vi "lvssh2_session_callback_send_32.vi"(4 "lvssh2_session_callback_send_function":refnum<vi>, 5 "Event Data":T1, 6 "User Event Ref":refnum<user-event>, 7 "Event Common Data":T3 {"Event Source" items=["LabVIEW UI"=0, "ActiveX"=1, "User Event"=25]}) -> ()   [LabVIEW 2013, in "libssh2.lvlib"]
uses:
  libssh2.lvlib
  <vilib>/event_ctls.llb/eventsource.ctl
  lvssh2_session_callback_send_function_input_args_32.ctl
  lvssh2_extensions.dll
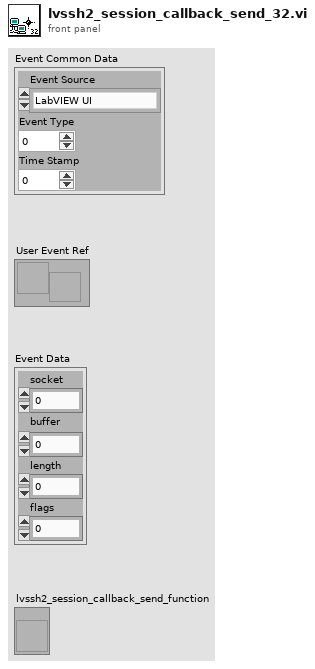
[diagram p1: front panel]
types:
  T1 = typedef "libssh2.lvlib/lvssh2_session_callback_send_function_input_args_32.ctl" = cluster{"socket":u32, "buffer":u32, "length":u32, "flags":i32}
  T2 = typedef "eventsource.ctl" = u32
  T3 = cluster{"Event Source":T2, "Event Type":u32, "Time Stamp":u32}
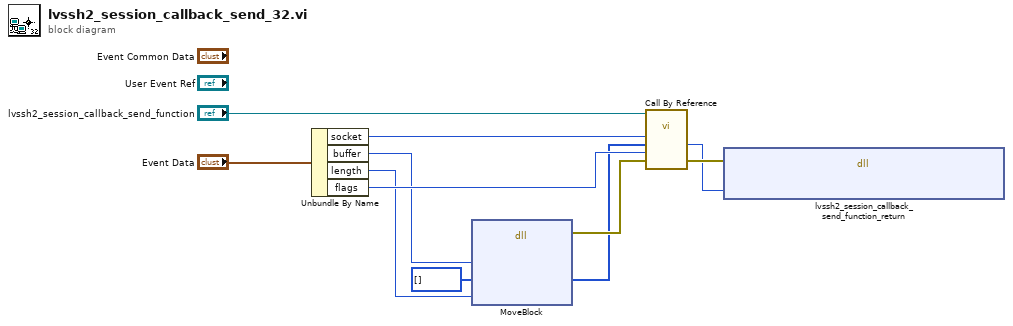
[diagram p0: block diagram]
diagram:
  n1 = Unbundle By Name("Event Data") -> ("socket"=w9:u32, "buffer"=w5:u32, "length"=w4:u32, "flags"=w8:i32)
  n2 = dll-call lib="LabVIEW" fn="MoveBlock"("ps"=w5, "pd"=u8[] [], "size"=w4) -> (error out=w3:errorcluster, "pd"=w1:u8[])  [unwired: 6 in, 1 out]
  n3 = call-by-ref "?"(reference="lvssh2_session_callback_send_function", "error in (no error)"=w3, "flags"=w8, "buffer"=w1, "socket"=w9) -> ("error out"=w7:errorcluster, "bytes send"=w6:i64)  [unwired: 7 in, 2 out]
  n4 = dll-call lib="C:/Users/pasca/Projects/Home/lvssh2/libssh2/lvssh2_extensions**.*" fn="lvssh2_session_callback_send_function_return"(error in=w7, "bytes_send"=w6) -> ()  [unwired: 4 in, 2 out]
